vi "prima_apl_v3.vi"() -> ()   [LabVIEW 2009]
panel:
  out "Dispozitiv de afisare 2":string
  out "Dispozitiv de afisare":string
  # "Prima aplicatie realizata in LabView"
  # "Aplicatia afiseaza un mesaj de bun venit in momentul cand este lansata\nsi mesajul \"Succes!\" dupa 500 de ms"
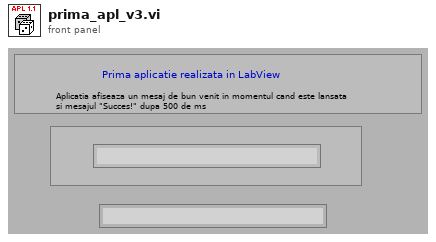
[diagram p1: front panel]
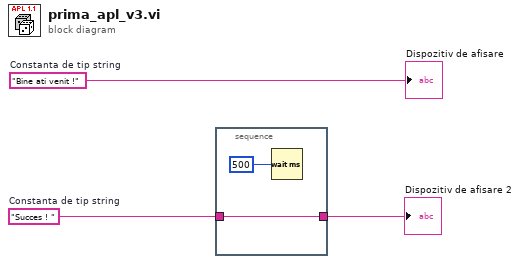
[diagram p0: block diagram]
diagram:
  w2 = "Succes ! "  # Constanta de tip string
  w3 = "Bine ati venit !"  # Constanta de tip string
  n1 = stacked-sequence {
    tunnel: w2 -> [w4]
    tunnel: [w4] -> w1
    frame #0 {
      n2 = Wait (ms)(milliseconds to wait=500) -> ()  [unwired: 1 out]
    }
  }
  "Dispozitiv de afisare 2" <- w1
  "Dispozitiv de afisare" <- w3
